vi "Inside_Entire_Space.vi"(2 "Model       Roll      Pitch       Yaw (deg)":sgl[](array[numeric])=[0.0, 0.0, 0.0] format="%#.2f", 3 "Current Position":sgl[](array[numeric])=[0.0, 200.0, 40.0] format="%.2f", 4 "Envelope":T1=[{"Max"=16000.0, "Min"=14000.0}, {"Max"=1000.0, "Min"=-1000.0}, {"Max"=700.0, "Min"=0.0}] {"Min" format="%#.1f"; "Max" format="%#.1f"}) -> (0 "Error Comments":string, 1 "Box Inside":bool)   [LabVIEW 2016]
uses:
  Box_size.ctl
  Globals/Preference_global.vi
panel:
  # "X                           Y                          Z"
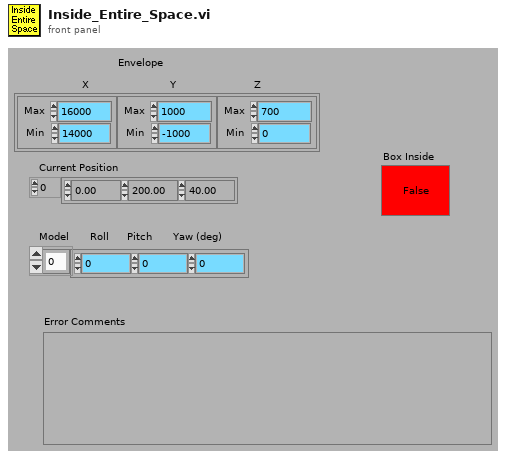
[diagram p1: front panel]
types:
  T1 = typedef "Box_size.ctl" = cluster{"Max":sgl, "Min":sgl}[]
  T2 = enum16{"To Traverse Coordinates", "To User Coordinates"}
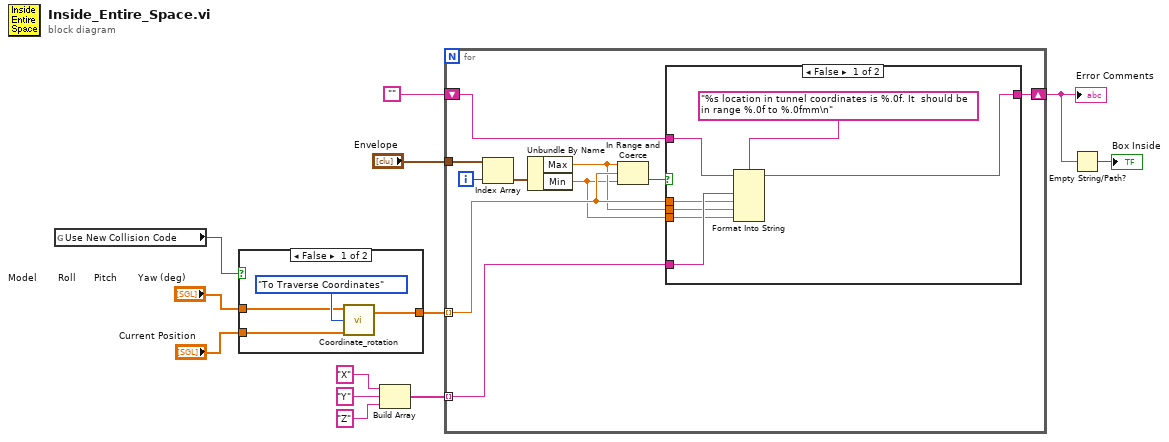
[diagram p0: block diagram]
diagram:
  n1 = global read "Preference_global.vi" "Use New Collision Code"() -> (w1:bool)
  n2 = case shown="False" w1 {
    tunnel: [w16 w17] -> w4
    tunnel: "Current Position" -> [w14 w17]
    tunnel: "Model       Roll      Pitch       Yaw (deg)" -> [w13 _]
    frame False {
      n3 = call "Coordinate_rotation.vi"("Roll-Pitch-Yaw"=w13, "Input Position"=w14, "Mode"=T2."To Traverse Coordinates") -> ("Output Position"=w16:sgl[])  [unwired: 2 in, 1 out]
    }
    frame True {
    }
  }
  n4 = Build Array("X", "Y", "Z") -> (w8:string[])
  n5 = for {
    shift-left: "" -> [w25]
    shift-right: [w26] -> w5
    tunnel: "Envelope" -> [w27]
    tunnel: w4 -> [w20] mode=indexing
    tunnel: w8 -> [w22] mode=indexing
    i -> [w23]
    n6 = Index Array(array=w27, index=w23) -> (element=w24:cluster{"Max":sgl, "Min":sgl})
    n7 = Unbundle By Name(w24) -> ("Max"=w19:sgl, "Min"=w18:sgl)
    n8 = In Range and Coerce(upper limit=w19, x=w20, lower limit=w18) -> (In Range?=w21:bool)  [unwired: 1 out]
    n9 = case shown="False" w21 {
      tunnel: w25 -> [w33 w35]
      tunnel: [w32 w35] -> w26
      tunnel: w22 -> [w31 _]
      tunnel: w20 -> [w30 _]
      tunnel: w19 -> [w29 _]
      tunnel: w18 -> [w28 _]
      frame False {
        n10 = Format Into String(format string="%s location in tunnel coordinates is %.0f. It  should be in range %.0f to %.0fmm\n" ("Format String"), initial string=w33, w31, w30, w29, w28) -> (resulting string=w32:string)  [unwired: 1 in, 1 out]
      }
      frame True {
      }
    }
  }
  "Error Comments" <- w5
  n11 = Empty String/Path?(string/path=w5) -> (empty?=→"Box Inside":bool)
